vi "SerializeInsertSpectMeasurement.vi"(3 "error in (no error)":errorcluster, 4 "InsertSpectMeasurement":T1, 5 "LotData in":refnum<class "LotData.lvclass">) -> (0 "error out":errorcluster, 1 "Json":string, 2 "LotData out":refnum<class "LotData.lvclass">)   [LabVIEW 2012, in "LotData.lvclass"]
uses:
  LotData.lvclass
  Controls/JsonTypes/InsertSpectrumMeasurement.ctl
  Controls/MeasurementType.ctl
  <vilib>/LVH/i3 JSON/JSON Generation/Create Value Files/Create Value - Object.vi
  <vilib>/LVH/i3 JSON/JSON Generation/Add Object Parameter Files/Add Object Parameter - String.vi
  <vilib>/LVH/i3 JSON/JSON Generation/Add Object Parameter Files/Add Object Parameter - Numeric.vi
  <vilib>/LVH/i3 JSON/JSON Generation/Add Object Parameter Files/Add Object Parameter - 1D Array Double.vi
  <vilib>/LVH/i3 JSON/i3-json.lvlib
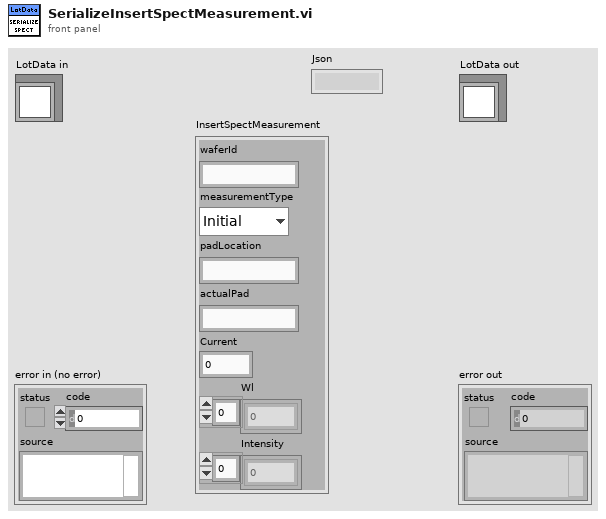
[diagram p1: front panel]
types:
  T1 = typedef "InsertSpectrumMeasurement.ctl" = cluster{"waferId":string, "measurementType":T2, "padLocation":string, "actualPad":string, "Current":dbl, "Wl":dbl[], "Intensity":dbl[]}
  T2 = typedef "MeasurementType.ctl" = enum16{"Initial", "Final"}
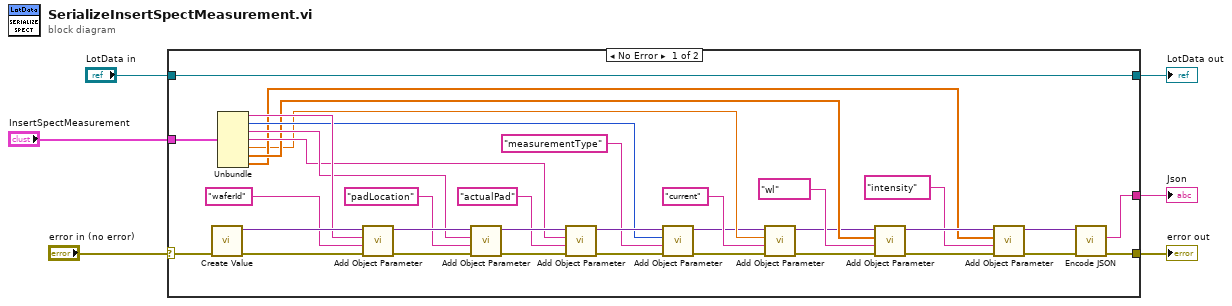
[diagram p0: block diagram]
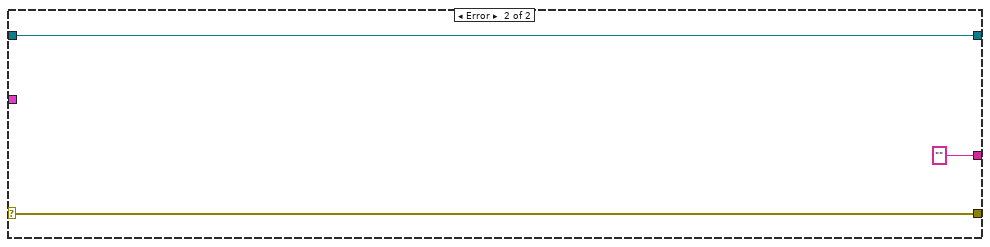
[diagram p2: hidden frame]
diagram:
  n1 = case shown="No Error" "error in (no error)" {
    selector: "error in (no error)" -> [w40 w44]
    tunnel: [w21 w44] -> w5
    tunnel: [w41 w43] -> w3
    tunnel: "LotData in" -> [w41 w43]
    tunnel: "InsertSpectMeasurement" -> [w35 _]
    tunnel: [w20 "" ("String")] -> w2
    frame No Error {
      n2 = call-poly <vilib>:"Create Value.vi"("error in (no error)"=w40) -> ("error out"=w38:errorcluster, "JSON Tree"=w39:variant)  [unwired: 9 in]
      n3 = Unbundle(w35) -> ("waferId"=w34:string, "measurementType"=w19:T2, "padLocation"=w26:string, "actualPad"=w17:string, "Current"=w10:dbl, "Wl"=w14:dbl[], "Intensity"=w13:dbl[])
      n4 = call-poly <vilib>:"Add Object Parameter.vi"("error in (no error)"=w38, "Name"="waferId", "String"=w34, "JSON Tree in (JSON Object)"=w39) -> ("error out"=w29:errorcluster, "JSON Tree out (JSON Object)"=w37:variant)  [unwired: 6 in]
      n5 = call-poly <vilib>:"Add Object Parameter.vi"("error in (no error)"=w29, "Name"="padLocation", "String"=w26, "JSON Tree in (JSON Object)"=w37) -> ("error out"=w30:errorcluster, "JSON Tree out (JSON Object)"=w36:variant)  [unwired: 6 in]
      n6 = call-poly <vilib>:"Add Object Parameter.vi"("error in (no error)"=w30, "Name"="actualPad", "String"=w17, "JSON Tree in (JSON Object)"=w36) -> ("error out"=w18:errorcluster, "JSON Tree out (JSON Object)"=w33:variant)  [unwired: 6 in]
      n7 = call-poly <vilib>:"Add Object Parameter.vi"("error in (no error)"=w18, "Name"="measurementType", "Numeric"=w19, "JSON Tree in (JSON Object)"=w33) -> ("error out"=w11:errorcluster, "JSON Tree out (JSON Object)"=w9:variant)  [unwired: 6 in]
      n8 = call-poly <vilib>:"Add Object Parameter.vi"("error in (no error)"=w11, "Name"="current", "Numeric"=w10, "JSON Tree in (JSON Object)"=w9) -> ("error out"=w7:errorcluster, "JSON Tree out (JSON Object)"=w8:variant)  [unwired: 6 in]
      n9 = call-poly <vilib>:"Add Object Parameter.vi"("error in (no error)"=w7, "Name"="wl", "1D Double"=w14, "JSON Tree in (JSON Object)"=w8) -> ("error out"=w22:errorcluster, "JSON Tree out (JSON Object)"=w25:variant)  [unwired: 6 in]
      n10 = call-poly <vilib>:"Add Object Parameter.vi"("error in (no error)"=w22, "Name"="intensity", "1D Double"=w13, "JSON Tree in (JSON Object)"=w25) -> ("error out"=w15:errorcluster, "JSON Tree out (JSON Object)"=w16:variant)  [unwired: 6 in]
      n11 = call <vilib>:"Encode JSON.vi"("error in (no error)"=w15, "JSON Tree"=w16) -> ("error out"=w21:errorcluster, "String"=w20:string)  [unwired: 4 in]
    }
    frame Error {
    }
  }
  "error out" <- w5
  "LotData out" <- w3
  "Json" <- w2
